vi "AmmeterComm.vi"() -> ()   [LabVIEW 2010]
uses:
  BaudRate.ctl
  VarableID.ctl
  AmmeterGlobalCostants.vi
panel:
  out "测量变量显示 2":dbl[][](graph)
  in  "视在功率":bool=TRUE
  in  "功率因数":bool=TRUE
  in  "电压":bool=TRUE
  in  "电流":bool=TRUE
  in  "退出系统":bool
  in  "软件使用说明":bool
  in  "启动采集":bool=TRUE
  in  "baud rate":T1=2400 caption="波特率" items=["1200"=1200, "2400"=2400, "4800"=4800, "9600"=9600, "19200"=19200, "38400"=38400, "115200"=115200, ""=0]
  out "测量变量显示":dbl[][](graph)
  # "智能电表信息采集系统"
  # "信号采集选项"
  # "端口参数设置"
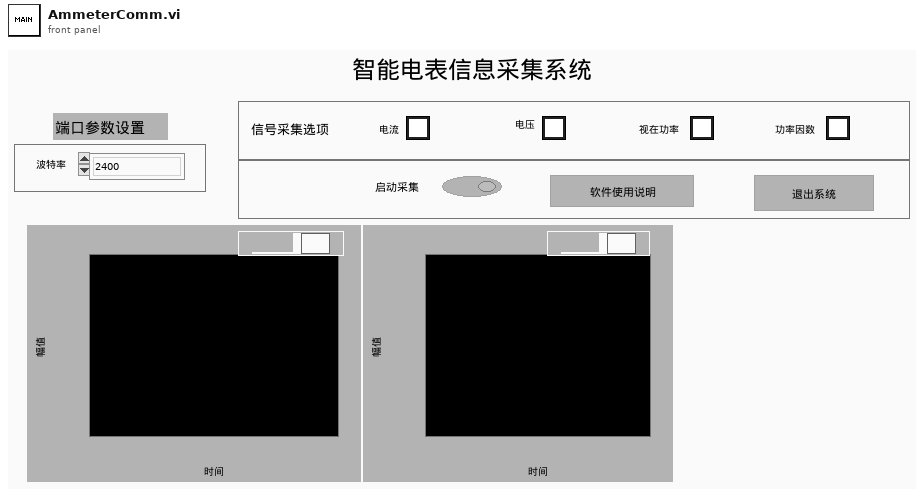
[diagram p1: front panel]
types:
  T1 = typedef "BaudRate.ctl" = u32
  T2 = typedef "OutputDataFormat.ctl" = cluster{"property":string, "dataIdentity":string, "value":string, "address":string, "timeStamp":string, "unit":string}
  T3 = typedef "VarableID.ctl" = enum16{"current", "voltage", "power", "PF"}
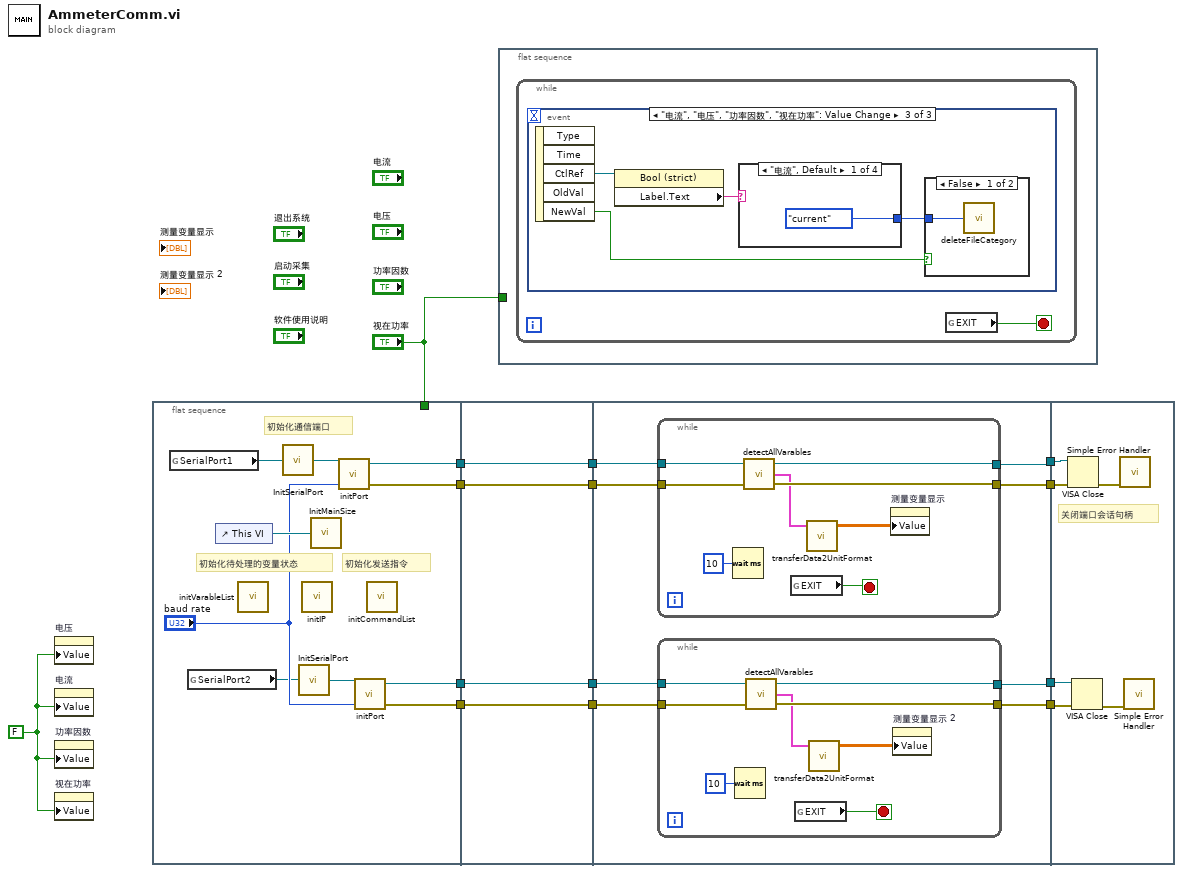
[diagram p0: block diagram]
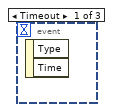
[diagram p2: hidden frame]
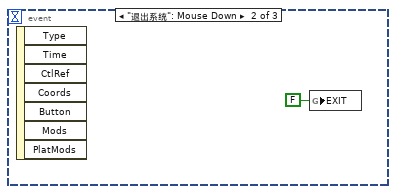
[diagram p3: hidden frame]
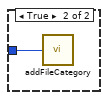
[diagram p4: hidden frame]
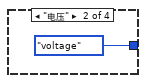
[diagram p5: hidden frame]
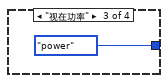
[diagram p6: hidden frame]
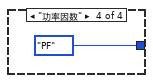
[diagram p7: hidden frame]
diagram:
  w7 = FALSE
  n1 = property on="电压" class="Bool (strict)"("Value"=w7) -> ()  [unwired: 2 in, 2 out]
  n2 = property on="电流" class="Bool (strict)"("Value"=w7) -> ()  [unwired: 2 in, 2 out]
  n3 = property on="功率因数" class="Bool (strict)"("Value"=w7) -> ()  [unwired: 2 in, 2 out]
  n4 = property on="视在功率" class="Bool (strict)"("Value"=w7) -> ()  [unwired: 2 in, 2 out]
  n5 = flat-sequence {
    tunnel: [w23] -> w10
    tunnel: "视在功率" -> [_]
    tunnel: [w24] -> w9
    tunnel: [w19] -> w5
    tunnel: [w18] -> w3
    tunnel: [w28] -> w11
    tunnel: w10 -> [w27]
    tunnel: w9 -> [w28]
    tunnel: [w27] -> w8
    tunnel: [w26] -> w6
    tunnel: w5 -> [w26]
    tunnel: [w25] -> w4
    tunnel: w3 -> [w25]
    tunnel: w11 -> [w36]
    tunnel: [w35] -> w14
    tunnel: [w34] -> w13
    tunnel: w8 -> [w33]
    tunnel: w6 -> [w32]
    tunnel: w4 -> [w31]
    tunnel: [w30] -> w2
    tunnel: [w29] -> w1
    tunnel: w14 -> [w57]
    tunnel: w13 -> [w56]
    tunnel: w2 -> [w54]
    tunnel: w1 -> [w53]
    frame #0 {
      # "初始化发送指令"
      # "初始化通信端口"
      # "初始化待处理的变量状态"
      n6 = global read "AmmeterGlobalCostants.vi" "SerialPort1"() -> (w16:refnum<visa-resource-name>)
      n7 = global read "AmmeterGlobalCostants.vi" "SerialPort2"() -> (w15:refnum<visa-resource-name>)
      n8 = control-ref of="This VI"() -> (w21:refnum<vi>)
      n9 = call "initVarableList.vi"() -> ()  [unwired: 12 in]
      n10 = call "InitSerialPort.vi"("default resource name"=w16) -> ("VISA resource name out"=w22:refnum<visa-resource-name>)
      n11 = call "InitSerialPort.vi"("default resource name"=w15) -> ("VISA resource name out"=w20:refnum<visa-resource-name>)
      n12 = call "initIP.vi"() -> ()  [unwired: 12 in]
      n13 = call "InitMainSize.vi"("VI Refnum In"=w21) -> ()  [unwired: 1 out]
      n14 = call "initPort.vi"("baud rate"="baud rate", "VISA resource name"=w22) -> ("error out"=w24:errorcluster, "reference out"=w23:refnum<visa-resource-name>)  [unwired: 2 in]
      n15 = call "initPort.vi"("baud rate"="baud rate", "VISA resource name"=w20) -> ("error out"=w18:errorcluster, "reference out"=w19:refnum<visa-resource-name>)  [unwired: 2 in]
      n16 = call "initCommandList.vi"() -> ()  [unwired: 12 in]
    }
    frame #1 {
    }
    frame #2 {
      n17 = while {
        tunnel: w36 -> [w49]
        tunnel: [w50] -> w35
        tunnel: [w52] -> w34
        tunnel: w33 -> [w51]
        stop <- w45 stop-if-true
        n18 = Wait (ms)(milliseconds to wait=u32 10) -> ()  [unwired: 1 out]
        n19 = call "detectAllVarables.vi"("error in (no error)"=w49, "VISA resource name"=w51) -> ("error out"=w52:errorcluster, "Data"=w48:T2[], "VISA resource name 2"=w50:refnum<visa-resource-name>)  [unwired: 1 in]
        n20 = global read "AmmeterGlobalCostants.vi" "EXIT"() -> (w45:bool)
        n21 = call "transferData2UnitFormat.vi"("Data"=w48) -> ("display"=w47:dbl[][])  [unwired: 4 in]
        n22 = property on="测量变量显示" class="WFChart (strict)"("Value"=w47) -> ()  [unwired: 2 in, 2 out]
      }
      n23 = while {
        tunnel: w31 -> [w41]
        tunnel: [w42] -> w30
        tunnel: [w44] -> w29
        tunnel: w32 -> [w43]
        stop <- w37 stop-if-true
        n24 = Wait (ms)(milliseconds to wait=u32 10) -> ()  [unwired: 1 out]
        n25 = call "detectAllVarables.vi"("error in (no error)"=w41, "VISA resource name"=w43) -> ("error out"=w44:errorcluster, "Data"=w40:T2[], "VISA resource name 2"=w42:refnum<visa-resource-name>)  [unwired: 1 in]
        n26 = global read "AmmeterGlobalCostants.vi" "EXIT"() -> (w37:bool)
        n27 = call "transferData2UnitFormat.vi"("Data"=w40) -> ("display"=w39:dbl[][])  [unwired: 4 in]
        n28 = property on="测量变量显示 2" class="WFChart (strict)"("Value"=w39) -> ()  [unwired: 2 in, 2 out]
      }
    }
    frame #3 {
      # "关闭端口会话句柄"
      n29 = VISA Close(VISA resource name=w57, error in (no error)=w56) -> (error out=w58:errorcluster)
      n30 = VISA Close(VISA resource name=w54, error in (no error)=w53) -> (error out=w55:errorcluster)
      n31 = call <vilib>:"Simple Error Handler.vi"("error in (no error)"=w58) -> ()  [unwired: 1 in, 8 out]
      n32 = call <vilib>:"Simple Error Handler.vi"("error in (no error)"=w55) -> ()  [unwired: 1 in, 8 out]
    }
  }
  n33 = flat-sequence {
    tunnel: "视在功率" -> [_]
    frame #0 {
      n34 = while {
        stop <- w59 stop-if-true
        n35 = event shown="[2] \"电流\", \"电压\", \"功率因数\", \"视在功率\": Value Change" {
          selector: _ -> [_ _ _]
          dyn-events: _ -> [_ _ _]
          timeout: _ -> [_ _ _]
          event Timeout {
            n36 = event-data() -> ()  [unwired: 1 in, 2 out]
          }
          event "退出系统": Mouse Down {
            n37 = event-data() -> ()  [unwired: 1 in, 7 out]
            n38 = global write "AmmeterGlobalCostants.vi" "EXIT"(FALSE ("EXIT")) -> ()
          }
          event "电流", "电压", "功率因数", "视在功率": Value Change {
            n39 = event-data() -> ("CtlRef"=w61:refnum<vi>, "NewVal"=w62:bool)  [unwired: 1 in, 3 out]
            n40 = property class="Bool (strict)"(reference=w61) -> ("Label.Text"=w64:string)  [unwired: 1 in, 2 out]
            n41 = case shown="\"电流\", Default" w64 {
              tunnel: [VarableID."current" ("VarableID") VarableID."voltage" ("VarableID") VarableID."power" ("VarableID") VarableID."PF" ("VarableID")] -> w63
              frame "电流", Default {
              }
              frame "电压" {
              }
              frame "视在功率" {
              }
              frame "功率因数" {
              }
            }
            n42 = case shown="False" w62 {
              tunnel: w63 -> [w65 w66]
              frame False {
                n43 = call "deleteFileCategory.vi"("VarableID"=w65) -> ()  [unwired: 1 in]
              }
              frame True {
                n44 = call "addFileCategory.vi"("VarableID"=w66) -> ()  [unwired: 1 in]
              }
            }
          }
        }
        n45 = global read "AmmeterGlobalCostants.vi" "EXIT"() -> (w59:bool)
      }
    }
  }
